vi "Initialize Default Registry.vi"(8 "error in (no error)":errorcluster) -> (0 "error out":errorcluster, 2 "Registry Name":string, 3 "Session Handle":T1)   [LabVIEW 2020, in "Registry.lvlib" / "Registry Session.lvclass"]
doc: "Creates a default registry, with the LabVIEW and Process collectors automatically added to it. This VI must be called before creating metrics or collectors that are registered in this registry.\n\nIt is generally recommended not to close the reference returned by this function during the application lifetime."
uses:
  Registry Session.lvclass
  Typedefs/Session Handle.ctl
  collector/LabVIEW collector/LabVIEW Collector.lvclass
  C:/Github-locals/PromVIEW/src/collector/collectable/Collectable.lvclass
  collector/process collector/Process Collector.lvclass
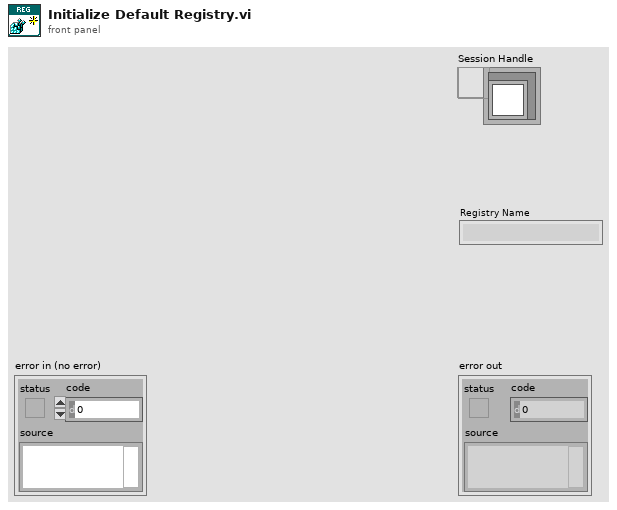
[diagram p1: front panel]
types:
  T1 = typedef "Registry.lvlib/Registry Session.lvclass/Session Handle.ctl" = refnum<data-value>
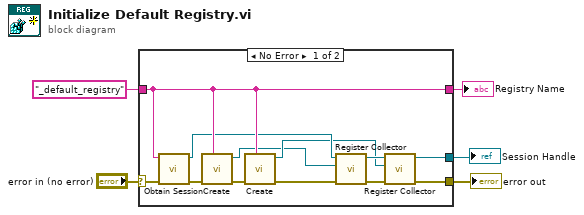
[diagram p0: block diagram]
diagram:
  n1 = case shown="No Error" "error in (no error)" {
    selector: "error in (no error)" -> [w15 w18]
    tunnel: [w6 w18] -> w4
    tunnel: "_default_registry" ("Session  Name ()") -> [w14 _]
    tunnel: [w14 _] -> w2
    tunnel: [w11 _] -> w1
    frame No Error {
      n2 = call "Obtain Session.vi"("error in (no error)"=w15, "Session  Name ()"=w14) -> ("error out"=w16:errorcluster, "Session Handle"=w13:T1)  [unwired: 8 in]
      n3 = call "Create.vi"("Registry Name"=w14, "error in (no error)"=w16) -> ("error out"=w17:errorcluster, "LabVIEW Collector out"=w9:refnum<class "LabVIEW Collector.lvclass">)  [unwired: 8 in]
      n4 = call "Create.vi"("Registry Name"=w14, "error in (no error)"=w17) -> ("error out"=w8:errorcluster, "Process Collector out"=w10:refnum<class "Process Collector.lvclass">)  [unwired: 8 in]
      n5 = call "Register Collector.vi"("error in (no error)"=w8, "Collector"=w9, "Session Handle in"=w13) -> ("error out"=w7:errorcluster, "Session Handle out"=w12:T1)  [unwired: 7 in]
      n6 = call "Register Collector.vi"("error in (no error)"=w7, "Collector"=w10, "Session Handle in"=w12) -> ("error out"=w6:errorcluster, "Session Handle out"=w11:T1)  [unwired: 7 in]
    }
    frame Error {
    }
  }
  "error out" <- w4
  "Registry Name" <- w2
  "Session Handle" <- w1
